vi "PopulatePortsAndSpeedsGain.vi"(9 "Ports and Speeds":refnum<vi>, 10 "Gain":refnum<vi>, 11 ".NET Refnum in":refnum<k24>) -> ()   [LabVIEW 2019]
uses:
  Dependencies/PVCamNET.dll
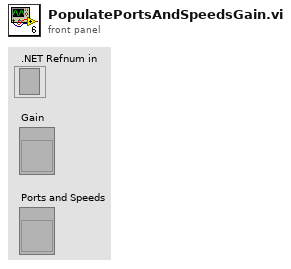
[diagram p1: front panel]
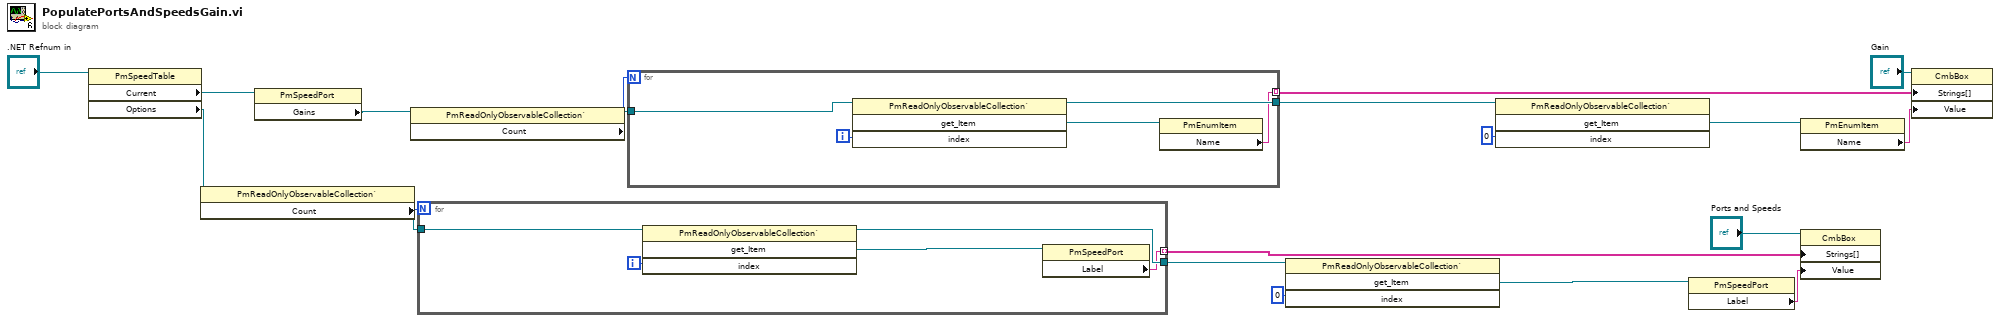
[diagram p0: block diagram]
diagram:
  n1 = property class="PmSpeedTable"(reference=".NET Refnum in") -> ("Current"=w2:refnum<k24>, "Options"=w11:refnum<k24>)  [unwired: 1 in, 2 out]
  n2 = property class="PmReadOnlyObservableCollection`"(reference=w11) -> (reference out=w12:refnum<k24>, "Count"=w13:i32)  [unwired: 1 in, 1 out]
  n3 = property class="PmSpeedPort"(reference=w2) -> ("Gains"=w3:refnum<k24>)  [unwired: 1 in, 2 out]
  n4 = property class="PmReadOnlyObservableCollection`"(reference=w3) -> (reference out=w5:refnum<k24>, "Count"=w4:i32)  [unwired: 1 in, 1 out]
  n5 = for {
    N: w13 -> [_]
    tunnel: w12 -> [w25]
    tunnel: [w23] -> w19
    tunnel: [w21] -> w15 mode=indexing
    i -> [w24]
    n6 = invoke class="PmReadOnlyObservableCollection`" method="get_Item"(reference=w25, "index"=w24) -> (reference out=w23:refnum<k24>, "get_Item"=w22:refnum<k24>)  [unwired: 2 in, 2 out]
    n7 = property class="PmSpeedPort"(reference=w22) -> ("Label"=w21:string)  [unwired: 1 in, 2 out]
  }
  n8 = for {
    N: w4 -> [_]
    tunnel: w5 -> [w30]
    tunnel: [w27] -> w8
    tunnel: [w26] -> w10 mode=indexing
    i -> [w29]
    n9 = invoke class="PmReadOnlyObservableCollection`" method="get_Item"(reference=w30, "index"=w29) -> (reference out=w27:refnum<k24>, "get_Item"=w28:refnum<k24>)  [unwired: 2 in, 2 out]
    n10 = property class="PmEnumItem"(reference=w28) -> ("Name"=w26:string)  [unwired: 1 in, 2 out]
  }
  n11 = invoke class="PmReadOnlyObservableCollection`" method="get_Item"(reference=w19, "index"=0) -> ("get_Item"=w17:refnum<k24>)  [unwired: 2 in, 3 out]
  n12 = invoke class="PmReadOnlyObservableCollection`" method="get_Item"(reference=w8, "index"=0) -> ("get_Item"=w7:refnum<k24>)  [unwired: 2 in, 3 out]
  n13 = property class="PmSpeedPort"(reference=w17) -> ("Label"=w16:string)  [unwired: 1 in, 2 out]
  n14 = property class="CmbBox"(reference="Ports and Speeds", "Strings[]"=w15, "Value"=w16) -> ()  [unwired: 1 in, 2 out]
  n15 = property class="PmEnumItem"(reference=w7) -> ("Name"=w20:string)  [unwired: 1 in, 2 out]
  n16 = property class="CmbBox"(reference="Gain", "Strings[]"=w10, "Value"=w20) -> ()  [unwired: 1 in, 2 out]
